vi "String combo refX.vi"(8 "error out":errorcluster, 11 "Ctrl ref":refnum<vi>[](array[refnum])) -> (0 "error out 2":errorcluster)   [LabVIEW 2022 SP3]
uses:
  Global 1.vi
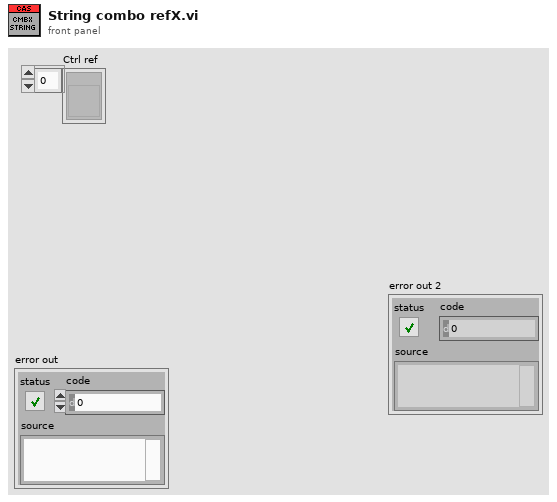
[diagram p1: front panel]
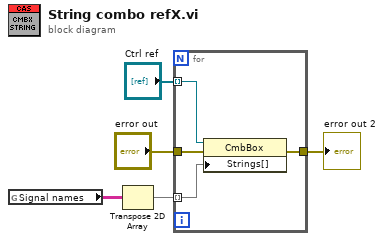
[diagram p0: block diagram]
diagram:
  n1 = global read "Global 1.vi" "Signal names"() -> (w2:string[][])
  n2 = Transpose 2D Array(2D array=w2) -> (transposed array=w1:string[][])
  n3 = for {
    tunnel: "Ctrl ref" -> [w9] mode=indexing
    tunnel: w1 -> [w6] mode=indexing
    tunnel: [w8] -> w3
    tunnel: "error out" -> [w7]
    n4 = property class="CmbBox"(reference=w9, error in=w7, "Strings[]"=w6) -> (error out=w8:errorcluster)  [unwired: 1 out]
  }
  "error out 2" <- w3
